vi "GoAndKickTacticCheckStateChange.vi"(8 "error in (no error)":errorcluster, 9 "Robot In":refnum<class "Robot.lvclass">, 10 "Game in":refnum<class "Game.lvclass">, 11 "GoAndKickTacticVSS in":refnum<class "GoAndKickTacticVSS.lvclass">) -> (0 "error out":errorcluster, 2 "States":enum16{"GoToBall", "Kick", "Exit"}(ring), 3 "GoAndKickTacticVSS out":refnum<class "GoAndKickTacticVSS.lvclass">)   [LabVIEW 2020, in "GoAndKickTacticVSS.lvclass"]
uses:
  GoAndKickTacticVSS.lvclass
  Game_class/Game.lvclass
  Robot_class/Robot.lvclass
  Game_class/Game.lvclass/Game.ctl
  Utilities_class/Utilities.lvclass
  Game_class/Read BallRef.vi
  Ball_class/Ball.lvclass
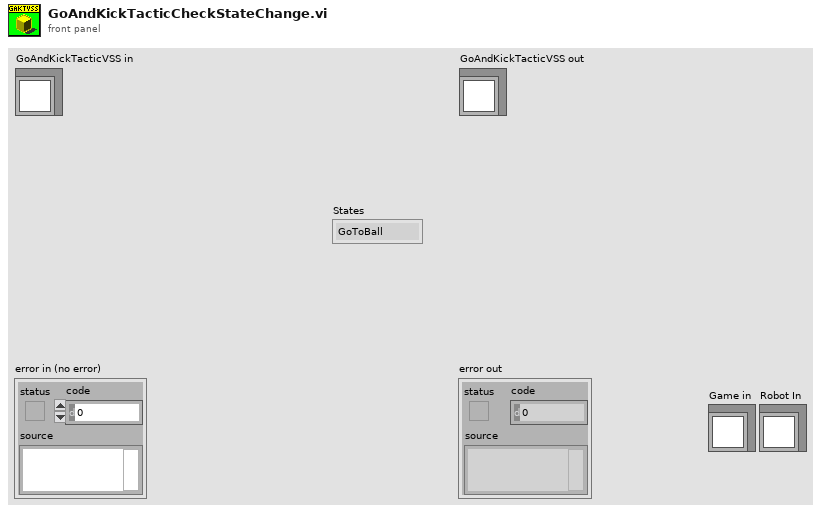
[diagram p1: front panel]
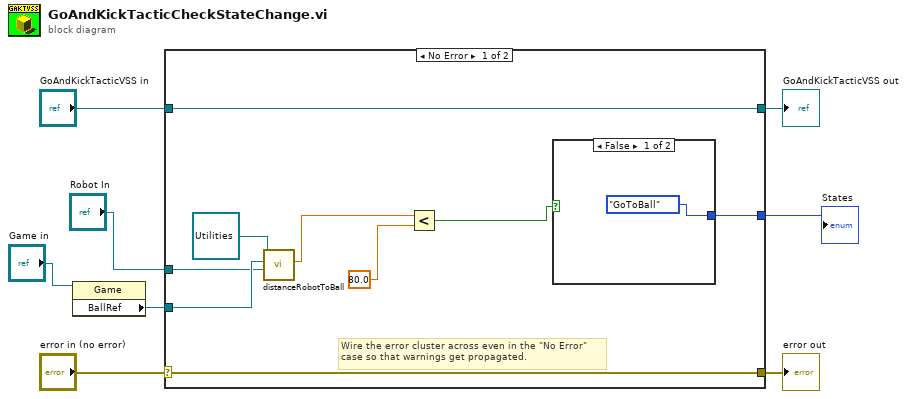
[diagram p0: block diagram]
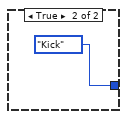
[diagram p2: hidden frame]
diagram:
  n1 = property class="Game"(reference="Game in") -> ("BallRef"=w2:refnum<class "Ball.lvclass">)  [unwired: 1 in, 2 out]
  n2 = case shown="No Error" "error in (no error)" {
    selector: "error in (no error)" -> [w16 w21]
    tunnel: [w16 w21] -> w7
    tunnel: [w17 w20] -> w5
    tunnel: "GoAndKickTacticVSS in" -> [w17 w20]
    tunnel: [w15 _] -> w4
    tunnel: w2 -> [w10 _]
    tunnel: "Robot In" -> [w9 _]
    frame No Error {
      # "Wire the error cluster across even in the \"No Error\"\ncase so that warnings get propagated."
      n3 = call "distanceRobotToBall.vi"("Robot"=w9, "Ball"=w10, "Utilities in"=refnum<class "Utilities.lvclass"> refnum) -> ("Distance Robot To Ball"=w13:dbl)  [unwired: 6 in, 2 out]
      n4 = Less?(x=w13, y=80.0) -> (x < y?=w11:bool)
      n5 = case shown="False" w11 {
        tunnel: [enum16{"GoToBall", "Kick", "Exit"}."GoToBall" ("States") enum16{"GoToBall", "Kick", "Exit"}."Kick" ("States")] -> w15
        frame False {
        }
        frame True {
        }
      }
    }
    frame Error {
    }
  }
  "error out" <- w7
  "GoAndKickTacticVSS out" <- w5
  "States" <- w4
